vi "Sub Super Duper_8_24_12a_JW.vi"(0 "VISA resource name":refnum<visa-resource-name>="GPIB0::17::INSTR", 1 "Sample Properties:":T6 {"Date Created" format="%<%Y/%m/%d>T"}, 2 "TRF Cluster":T7={"Step 4"=-38.0, "# of Loops"=1.0, "Transfer 2"=FALSE, "Start 4"=-2.0, "Total Points 2"=2, "Start 3"=40.0, "Stop 2"=-40.0, "Step 3"=-1.0, "Loop Step"=0.0, "Integration Time 3"=0, "Loop Wait"=0.0, "First Step"=0.0} {"Loop Wait" format="%<%H:%M:%S>t"; "Integration Time 3" scale=0.0..2.0; "Step 3" format="%.2f"; "Stop 2" format="%.2f"; "Start 3" format="%.2f"; "Start 4" format="%.2f"; "Step 4" format="%.2f"}, 3 "TSP Cluster":T8={"Transport"=FALSE, "Start 2"=0.0, "Stop 3"=-60.0, "Step 2"=-1.0, "Start"=0.0, "Step"=-10.0, "Total Points"=7, "Integration Time"=0} {"Integration Time" scale=0.0..2.0; "Step" format="%.2f"; "Start" format="%.2f"; "Step 2" format="%.2f"; "Stop 3" format="%.2f"; "Start 2" format="%.2f"}, 4 "Compliance Cluster":T3={"Var1 sweep settings"={"sweep spacing (linear: 0)"=0, "sweep mode"=FALSE, "compliance (V)"=100.0, "compliance (A)"=0.001}, "Var1 sweep settings 2"={"sweep spacing (linear: 0)"=0, "sweep mode"=FALSE, "compliance (V)"=100.0, "compliance (A)"=0.001}, "Var2 step settings 2"={"compliance (A)"=0.001, "compliance (V)"=100.0}, "Var2 step settings"={"compliance (A)"=0.001, "compliance (V)"=100.0}} {"Var2 step settings"."compliance (V)" format="%.2f"; "Var2 step settings"."compliance (A)" format="%^.2e"; "Var2 step settings 2"."compliance (V)" format="%.2f"; "Var2 step settings 2"."compliance (A)" format="%^.2e"; "Var1 sweep settings 2"."compliance (A)" format="%^.2e"; "Var1 sweep settings 2"."compliance (V)" format="%.2f"; "Var1 sweep settings 2"."sweep spacing (linear: 0)" items=["linear", "log 10", "log 25", "log 50"]; "Var1 sweep settings"."compliance (A)" format="%^.2e"; "Var1 sweep settings"."compliance (V)" format="%.2f"; "Var1 sweep settings"."sweep spacing (linear: 0)" items=["linear", "log 10", "log 25", "log 50"]}, 5 "error in":errorcluster, 6 "Saved Folder:":path=path "C:/1DATA/2011", 7 "Wait Cluster":T2 {"Wait Time (s)" format="%.1g"; "Wait Countdown" format="%<%H:%M:%S%1u>t"}, 9 "Stop \nCountdown":bool, 11 "Loop Count":dbl) -> (8 "Status Indicator":bool, 10 "Vt Cluster":T1 {"Id Max" format="%.3g"; "Vt Max" format="%.3g"; "Vt Min" format="%.3g"; "Vt Ratio" format="%.3g"}, 14 "VISA resource name out":refnum<visa-resource-name>, 15 "TRF Path":path, 16 "TSP Path":path, 17 "Graph Cluster":T4, 18 "Char Cluster":T5 {"Mobility-Lin" format="%#_4e"; "On/Off" format="%#_4e"; "Mobility-Sat" format="%#_4e"}, 19 "error out":errorcluster)   [LabVIEW 2012]
uses:
  <vilib>/Platform/TimedLoop/XDataNode/wakeup.ctl
  <vilib>/Platform/TimedLoop/XDataNode/XDNodeRunTimeDep.lvlib
  <vilib>/Platform/TimedLoop/XDataNode/nitl_modes.ctl
  <vilib>/Platform/TimedLoop/XDataNode/timing_clust.ctl
  <vilib>/Platform/TimedLoop/XDataNode/XDataNode.xnode
panel:
  # "Vg Sweep"
  # "Vd Step"
  # "Loops and Integration Time"
  # "Device Characteristics"
  # "Sample Properties:"
  # "%"
  # "nm"
  # "Device Properties:"
  # "um"
  # "um"
  # "Vg Step"
  # "Vd Step"
  # "Integration Time"
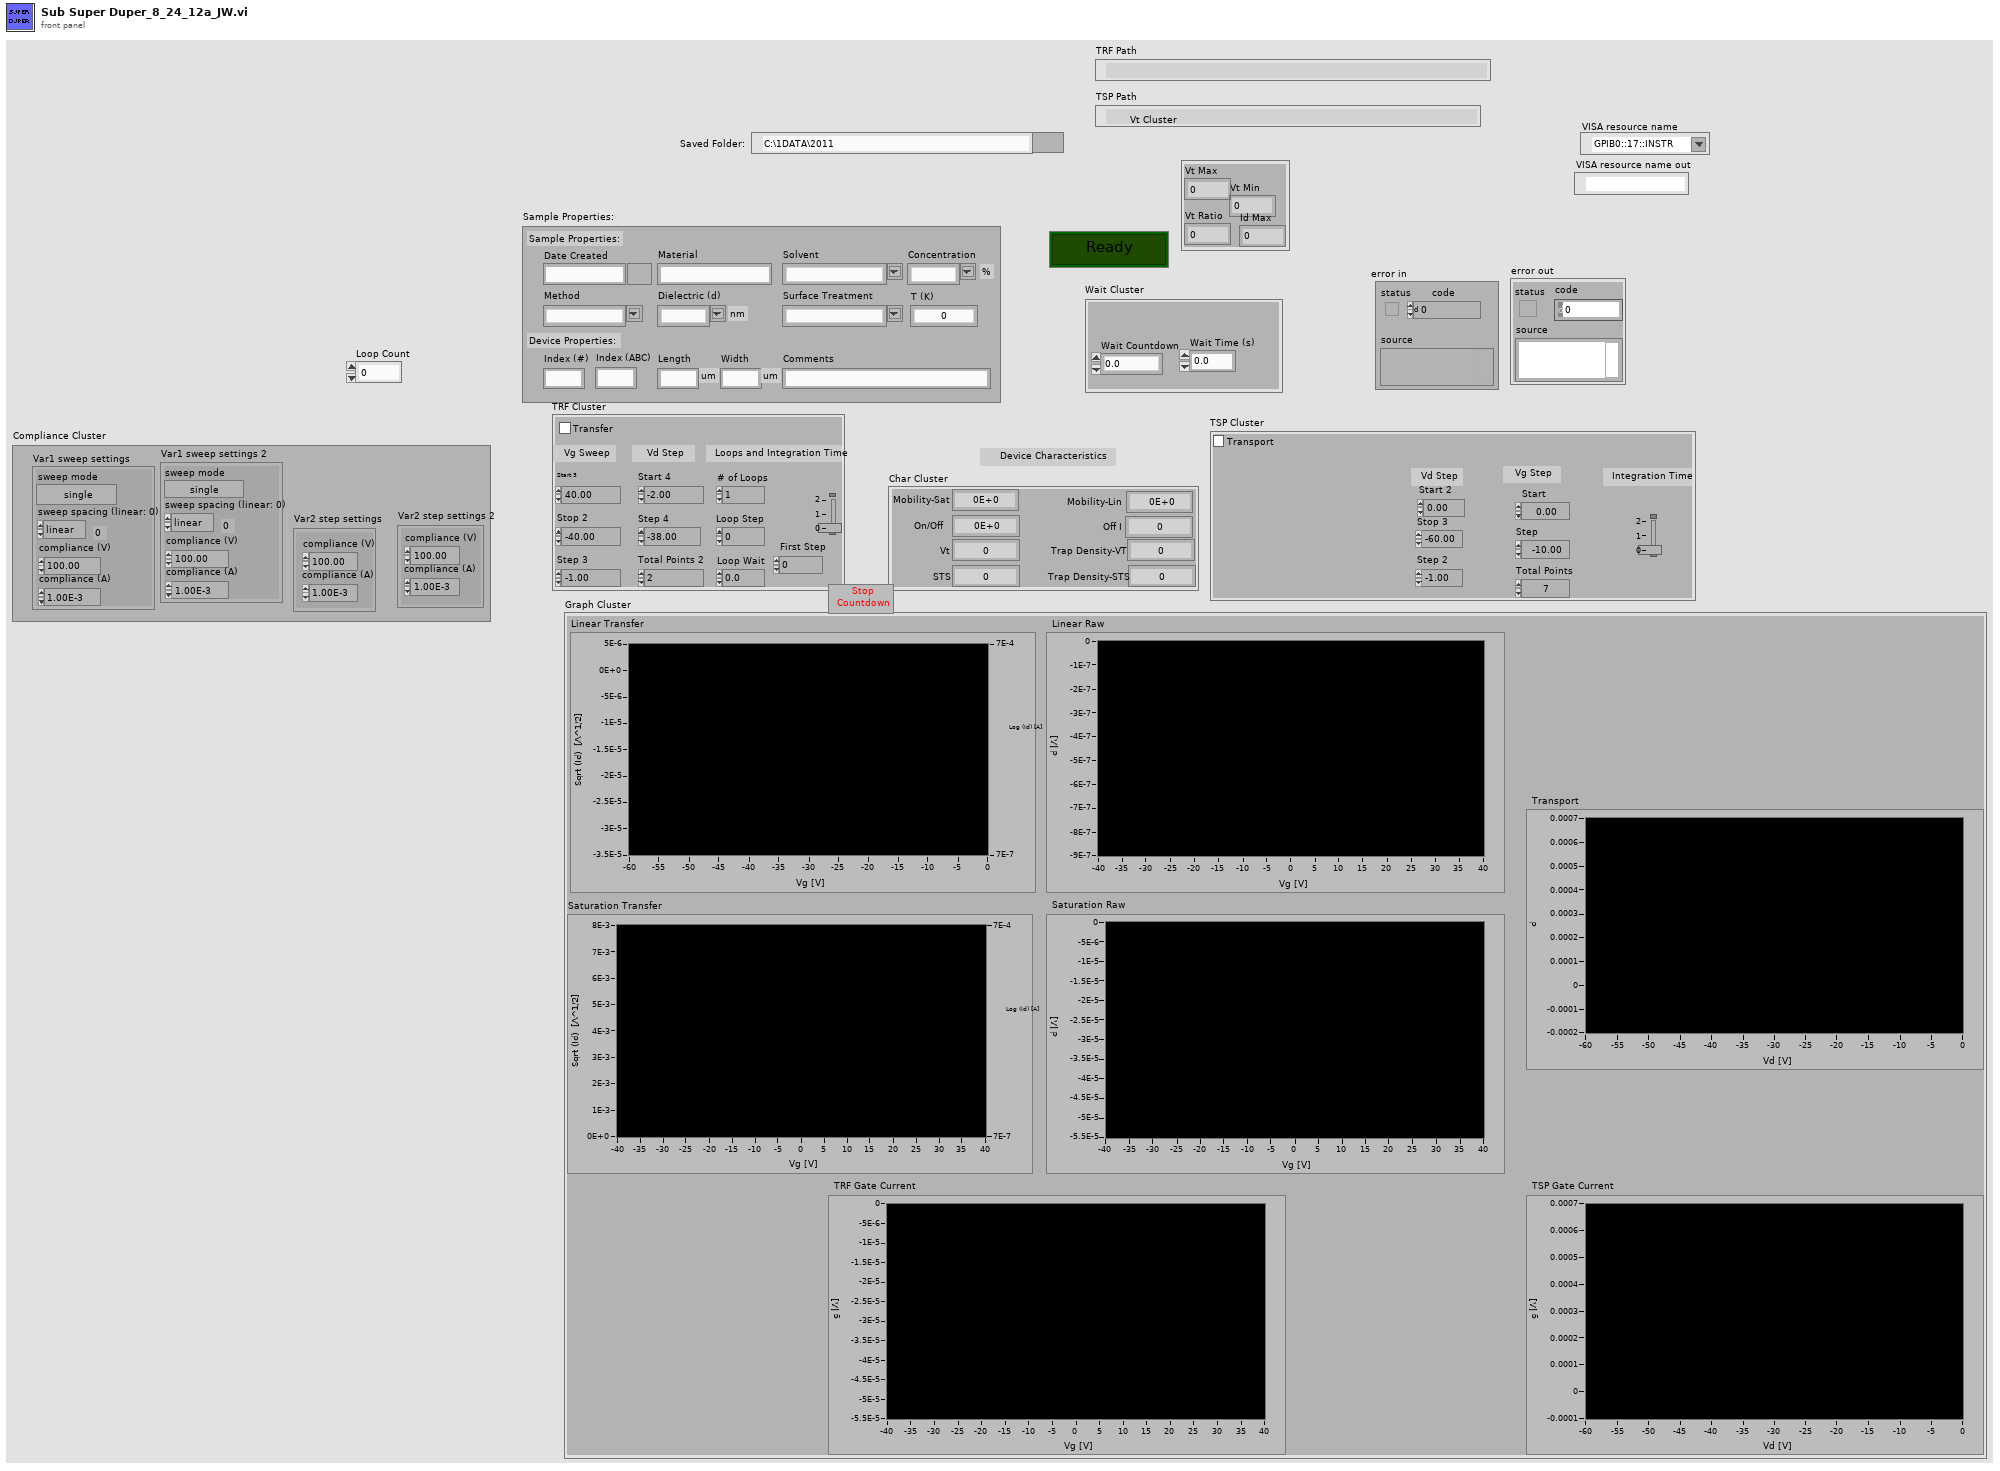
[diagram p1: front panel]
types:
  T1 = cluster{"Vt Max":i32, "Vt Min":i32, "Vt Ratio":i32, "Id Max":i32}
  T2 = cluster{"Wait Countdown":dbl, "Wait Time (s)":dbl}
  T3 = cluster{"Var1 sweep settings":cluster{"sweep spacing (linear: 0)":u16, "sweep mode":bool, "compliance (V)":dbl, "compliance (A)":dbl}, "Var1 sweep settings 2":cluster{"sweep spacing (linear: 0)":u16, "sweep mode":bool, "compliance (V)":dbl, "compliance (A)":dbl}, "Var2 step settings 2":cluster{"compliance (A)":dbl, "compliance (V)":dbl}, "Var2 step settings":cluster{"compliance (A)":dbl, "compliance (V)":dbl}}
  T4 = cluster{"Linear Transfer":cluster{dbl[], "trace":dbl[]}[], "Linear Raw":cluster{dbl[], dbl[]}[], "Saturation Transfer":cluster{dbl[], "trace":dbl[]}[], "Saturation Raw":cluster{dbl[], dbl[]}[], "Transport":cluster{dbl[], dbl[]}[], "TRF Gate Current":cluster{dbl[], dbl[]}[], "TSP Gate Current":cluster{dbl[], dbl[]}[]}
  T5 = cluster{"Mobility-Sat":dbl, "Mobility-Lin":dbl, "On/Off ":dbl, "Off I":dbl, "Vt":dbl, "STS":dbl, "Trap Density-VT":dbl, "Trap Density-STS":dbl}
  T6 = cluster{"Date Created":timestamp, "Material":string, "Solvent":string, "Concentration":string, "Method":string, "Dielectric (d)":string, "Index (#)":string, "Index (ABC)":string, "Length":string, "Width":string, "Surface Treatment":string, "Comments":string, "T (K)":dbl}
  T7 = cluster{"Step 4":dbl, "# of Loops":dbl, "Transfer 2":bool, "Start 4":dbl, "Total Points 2":u16, "Start 3":dbl, "Stop 2":dbl, "Step 3":dbl, "Loop Step":dbl, "Integration Time 3":u32, "Loop Wait":dbl, "First Step":dbl}
  T8 = cluster{"Transport":bool, "Start 2":dbl, "Stop 3":dbl, "Step 2":dbl, "Start":dbl, "Step":dbl, "Total Points":u16, "Integration Time":u32}
  T9 = typedef "XDNodeRunTimeDep.lvlib/timing_clust.ctl" = cluster{"Expected End [f-1]":u64, "Actual End [f-1]":u64, "Finished Late? [f-1]":bool, "Expected End [i-1]":u64, "Actual End [i-1]":u64, "Finished Late? [i-1]":bool, "Expected Start [i]":u64, "Actual Start [i]":u64, "Expected Start [f]":u64, "Actual Start [f]":u64, "Source Name":string, "Structure Name":string, "Period":i64, "Deadline":i64, "Offset":i64, "Start":i64, "Priority":i32, "Timeout":i32, "Mode":T10, "Wakeup Reason":T11, "Error":errorcluster, "Source Type":string, "Secondary Source Type":string, "Global End Time":u64, "Global Start Time":u64, "Frame Duration":u64, "Iteration Duration":u64, "Assigned CPU":i32, "I/O Scan Engine Mode":u32}
  T10 = typedef "XDNodeRunTimeDep.lvlib/nitl_modes.ctl" = enum32{"No Change", "Process missed periods, maintain original phase", "Discard missed periods, maintain original phase", "Process missed periods, ignore original phase", "Discard missed periods, ignore original phase"}
  T11 = typedef "XDNodeRunTimeDep.lvlib/wakeup.ctl" = enum32{"Normal", "Aborted", "Asynchronous wakeup", "Timing source error", "Timed loop error", "Timeout"}
  T12 = cluster{"sweep spacing (linear: 0)":u16, "sweep mode":bool, "compliance (V)":dbl, "compliance (A)":dbl}
  T13 = cluster{"compliance (A)":dbl, "compliance (V)":dbl}
  T14 = cluster{"Start 3":dbl, "Stop 2":dbl, "Step 3":dbl, "sweep spacing (linear: 0)":u16, "sweep mode":bool, "compliance (V)":dbl, "compliance (A)":dbl}
  T15 = cluster{"compliance (A)":dbl, "compliance (V)":dbl, "Start 4":dbl, "Total Points 2":u16, dbl}
  T16 = cluster{"Vt Max":i32, "Vt Min":i32, "Vt Ratio":i32, "Id Max":dbl}
  T17 = cluster{"Mobility-Sat":dbl, "Mobility-Lin":dbl, "On/Off Current":dbl, "Off I":dbl, "Vt":dbl, "STS":dbl, "Trap Density-VT":dbl, "Trap Density-STS":dbl}
  T18 = cluster{"Linear Sqrt":cluster{dbl[], "trace":dbl[]}[], "Linear Log":cluster{dbl[], "trace":dbl[]}[], "Linear Raw":cluster{dbl[], dbl[]}[], "Saturation Sqrt":cluster{dbl[], "trace":dbl[]}[], "Saturation Log":cluster{dbl[], "trace":dbl[]}[], "Saturation Raw":cluster{dbl[], "trace":dbl[]}[], "Gate Current":cluster{dbl[], "trace":dbl[]}[]}
  T19 = cluster{"Start 2":dbl, "Stop 3":dbl, "Step 2":dbl, "sweep spacing (linear: 0)":u16, "sweep mode":bool, "compliance (V)":dbl, "compliance (A)":dbl}
  T20 = cluster{"compliance (A)":dbl, "compliance (V)":dbl, "Start":dbl, "Total Points":u16, "Step":dbl}
  T21 = cluster{"Transport":cluster{dbl[], dbl[]}[], "Gate Current":cluster{dbl[], dbl[]}[]}
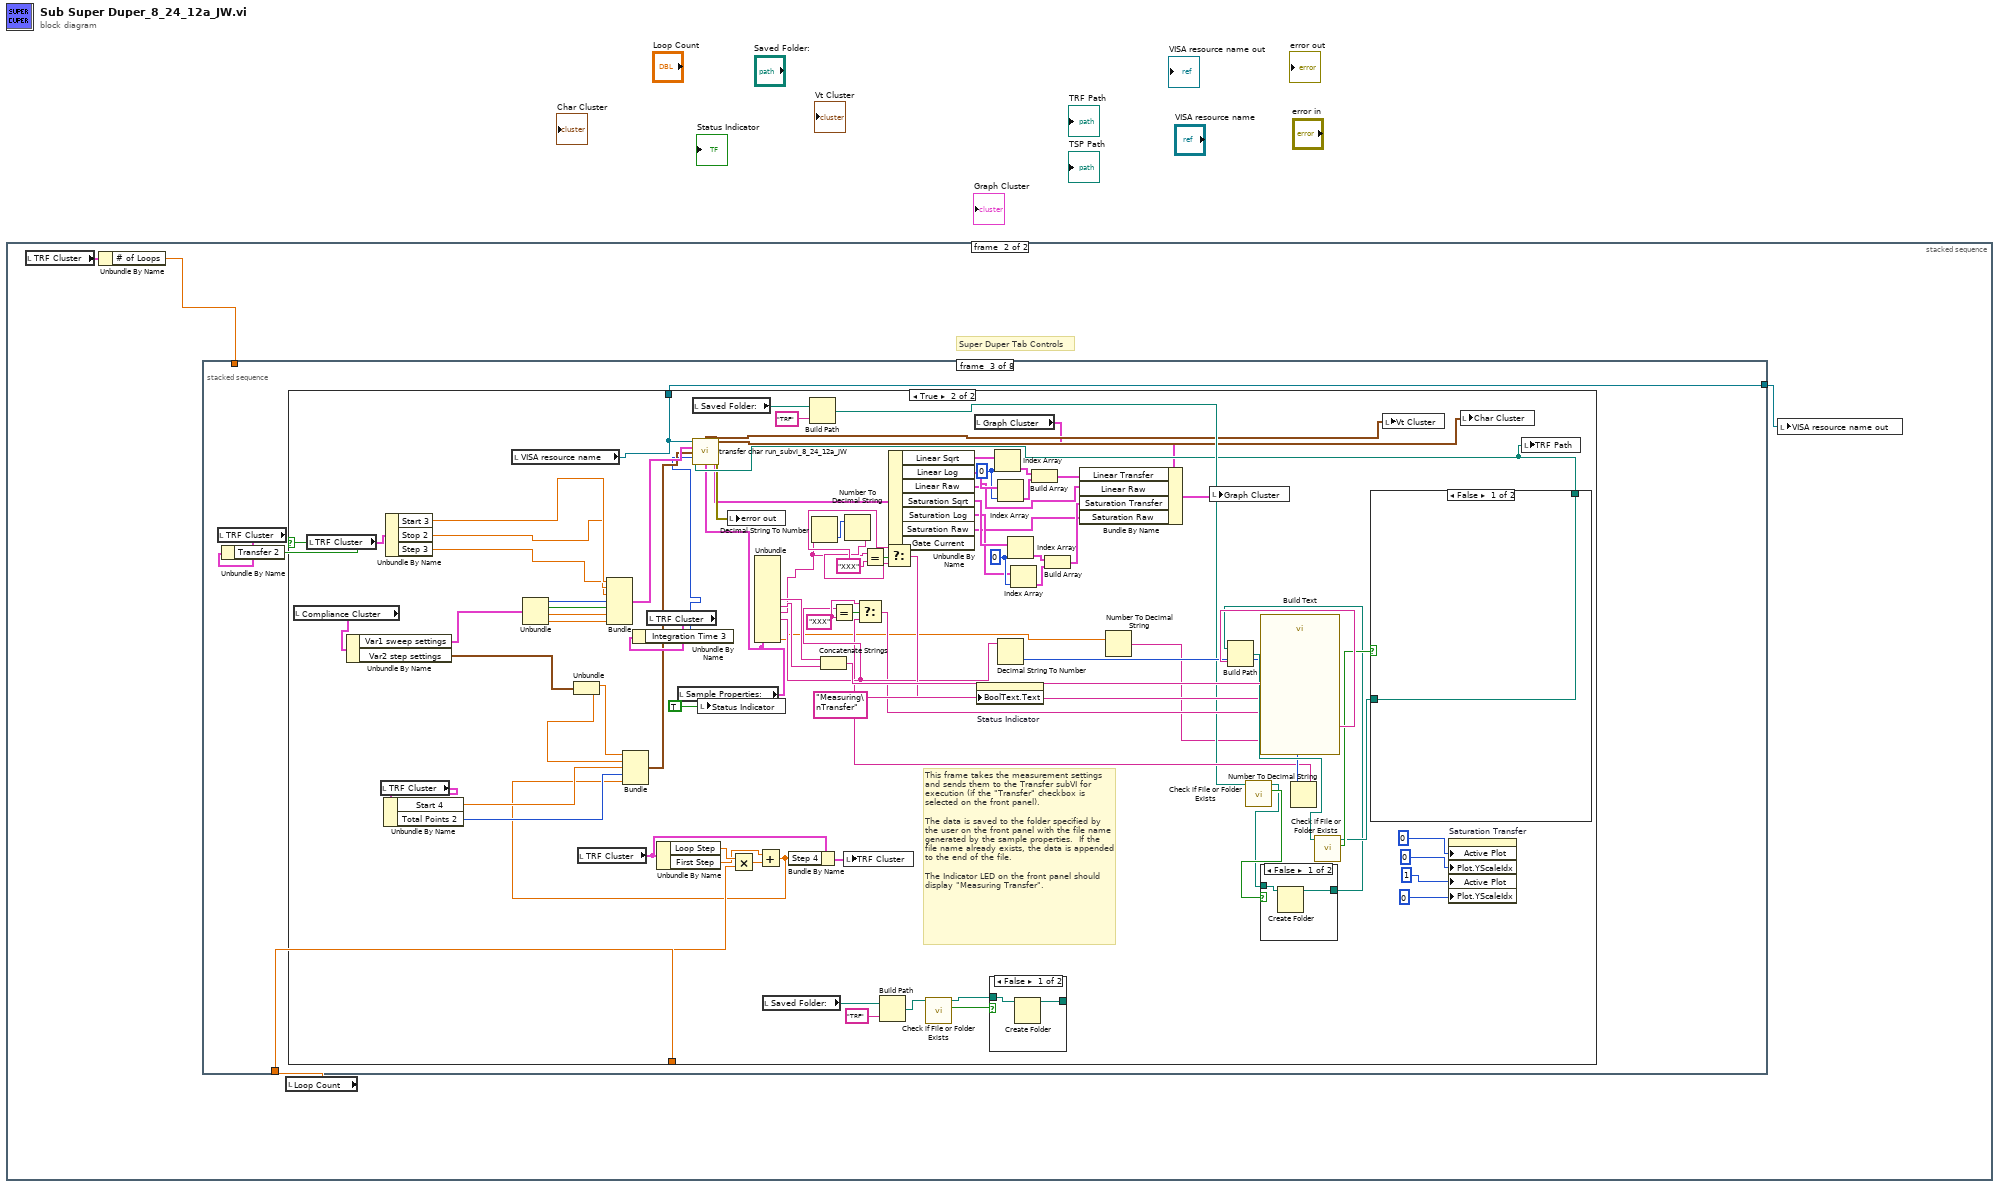
[diagram p0: block diagram]
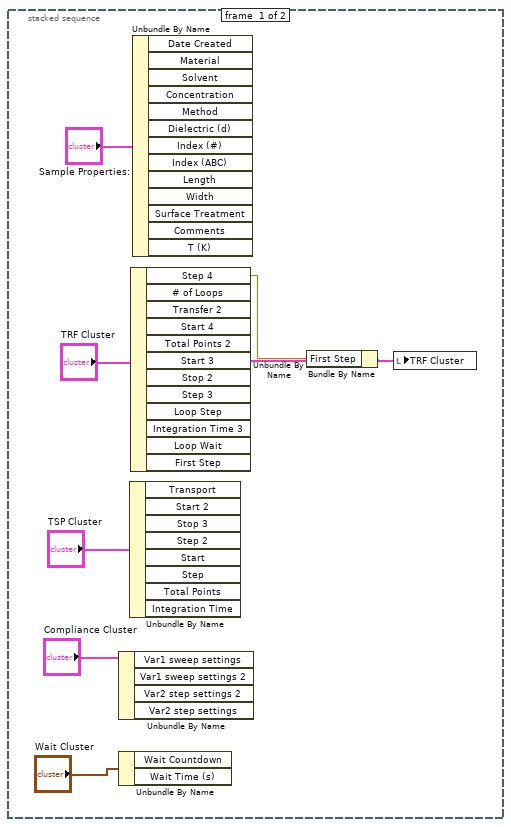
[diagram p2: hidden frame]
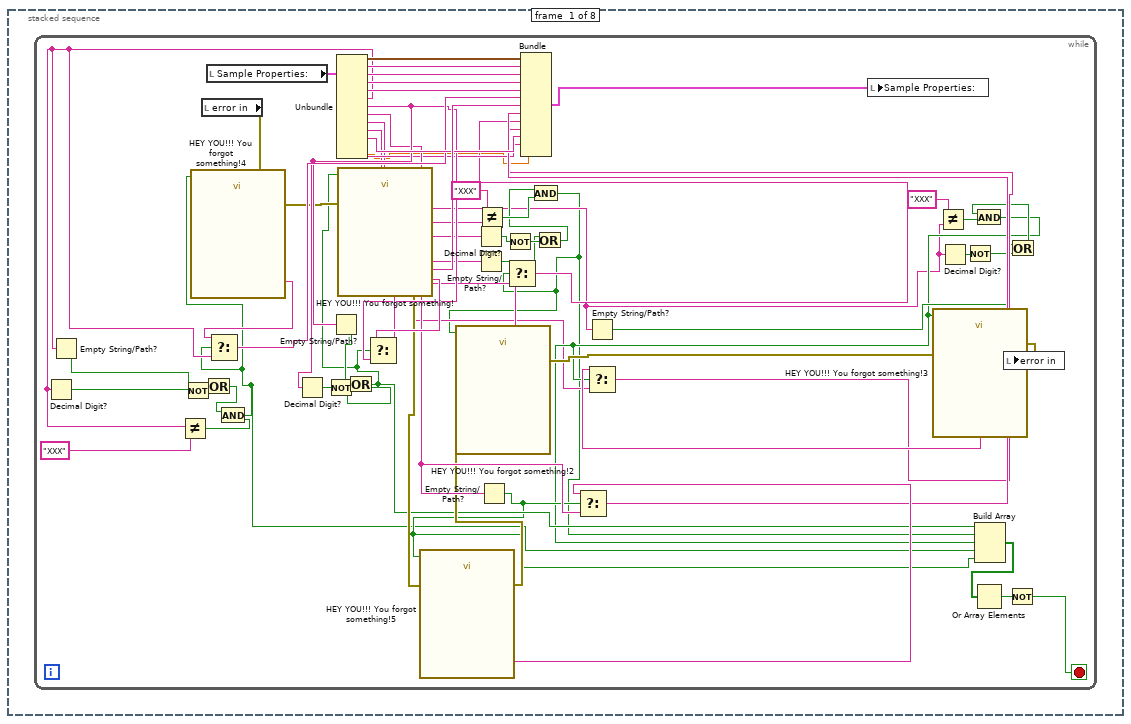
[diagram p3: hidden frame]
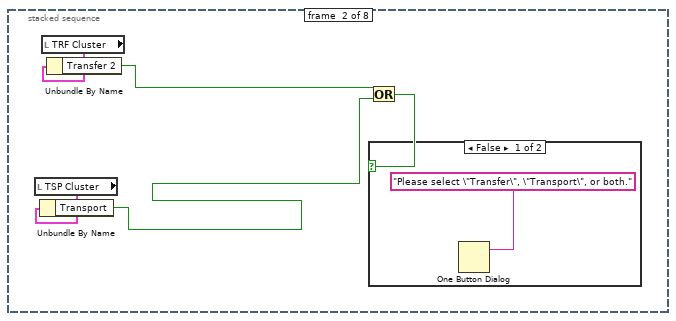
[diagram p4: hidden frame]
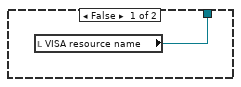
[diagram p6: hidden frame]
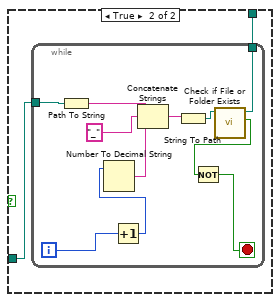
[diagram p9: hidden frame]
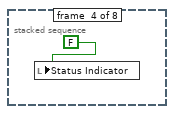
[diagram p10: hidden frame]
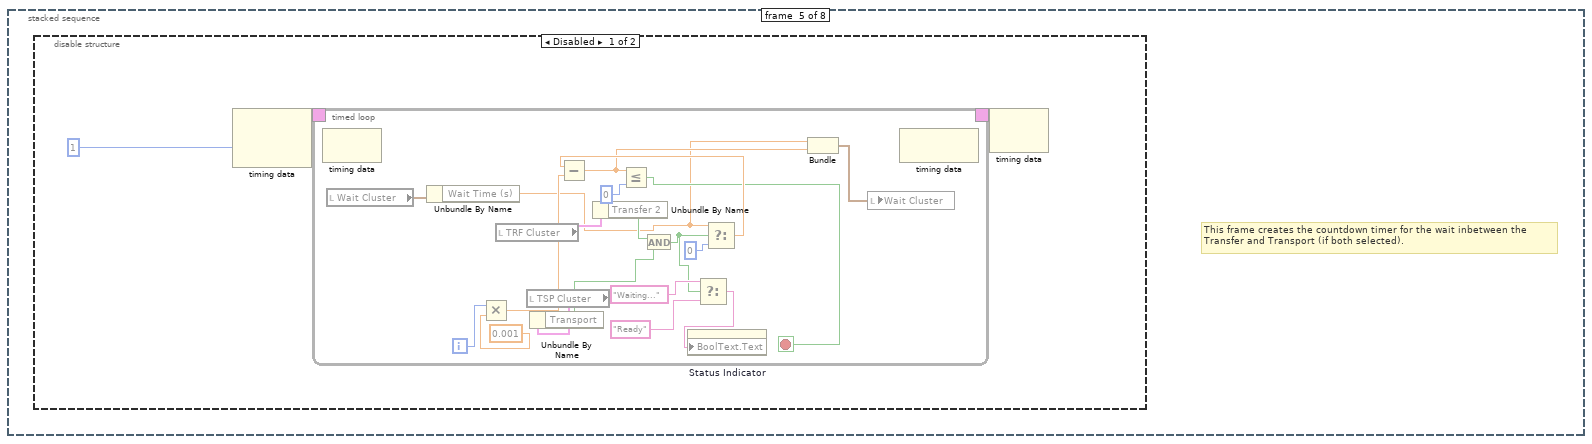
[diagram p11: hidden frame]
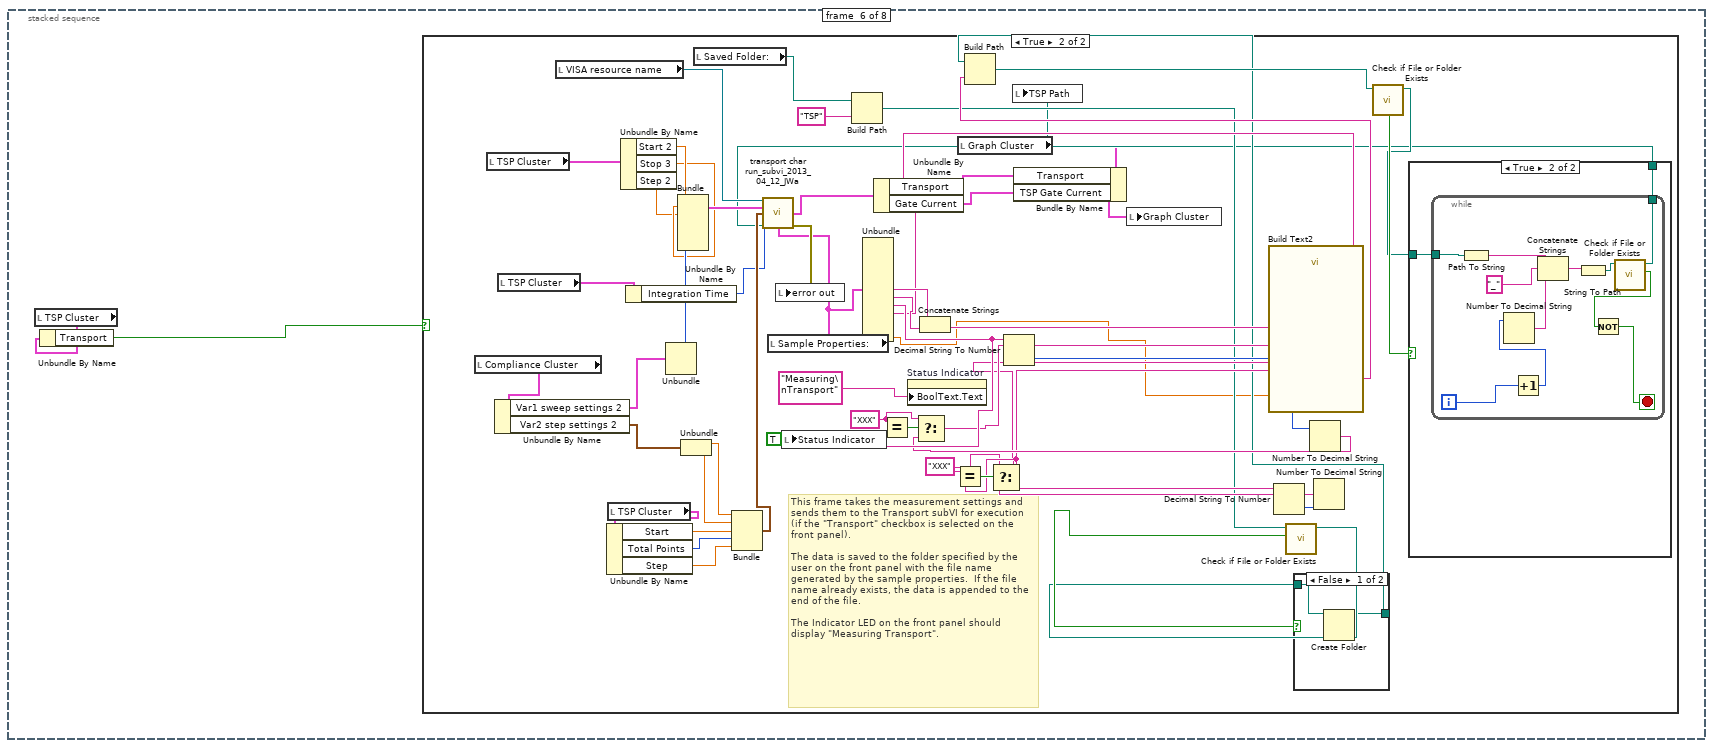
[diagram p13: hidden frame]
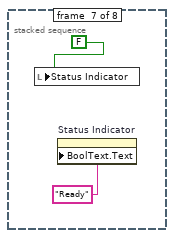
[diagram p17: hidden frame]
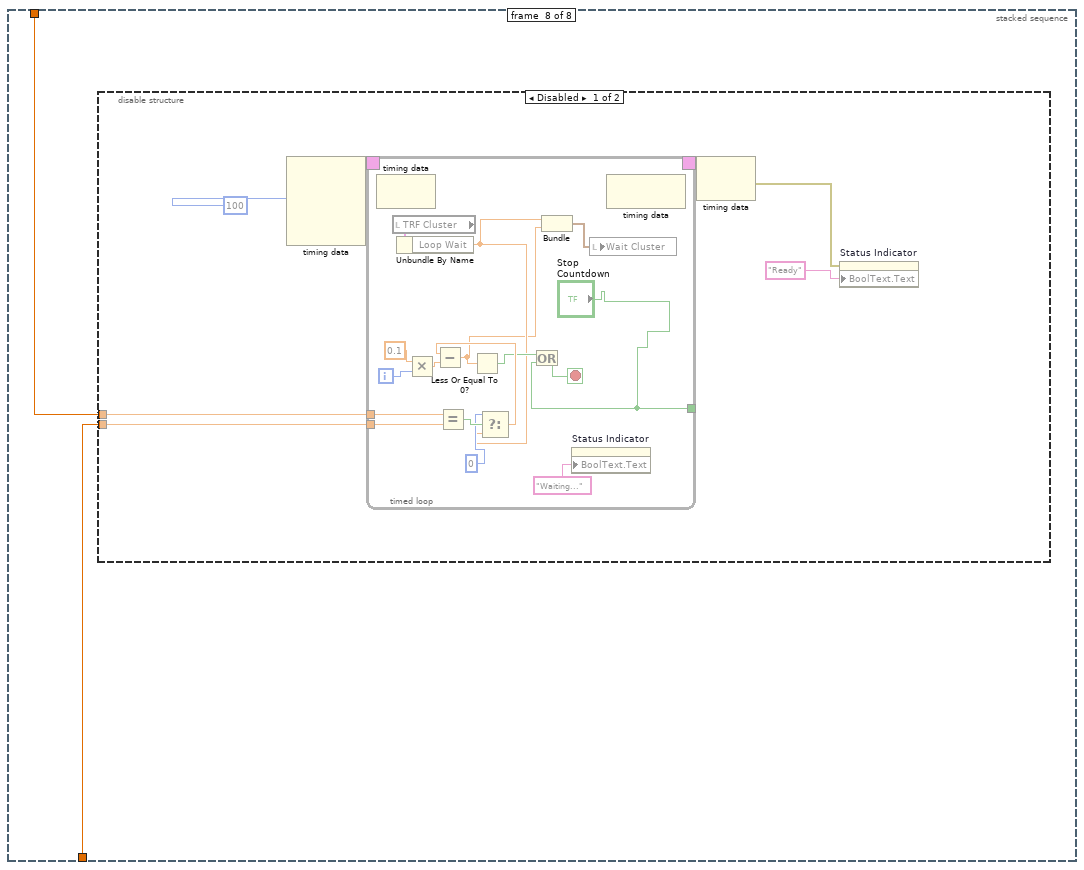
[diagram p18: hidden frame]
diagram:
  n1 = stacked-sequence {
    frame #0 {
      n2 = Unbundle By Name("Compliance Cluster") -> ()  [unwired: 4 out]
      n3 = Unbundle By Name("Wait Cluster") -> ()  [unwired: 2 out]
      n4 = Unbundle By Name("TSP Cluster") -> ()  [unwired: 8 out]
      n5 = Unbundle By Name("TRF Cluster") -> ("Step 4"=w7:dbl)  [unwired: 11 out]
      n6 = Unbundle By Name("Sample Properties:") -> ()  [unwired: 13 out]
      n7 = Bundle By Name(cluster="TRF Cluster", "First Step"=w7) -> (w5:T7)
      n8 = local write "TRF Cluster"(w5) -> ()
    }
    frame #1 {
      # "Super Duper Tab Controls"
      n9 = local read "TRF Cluster"() -> (w11:T7)
      n10 = Unbundle By Name(w11) -> ("# of Loops"=w10:dbl)
      n11 = local read "Loop Count"() -> (w8:dbl)
      n12 = stacked-sequence {
        tunnel: w8 -> [_ _ w81 _ _ _ _ w300]
        tunnel: w10 -> [_ _ _ _ _ _ _ w299]
        tunnel: [_ _ w78 _ _ _ _ _] -> w9
        frame #0 {
          n13 = while {
            stop <- w37 stop-if-true
            n14 = local read "error in"() -> (w43:errorcluster)
            n15 = local read "Sample Properties:"() -> (w66:T6)
            n16 = Unbundle(w66) -> ("Date Created"=w67:timestamp, "Material"=w68:string, "Solvent"=w69:string, "Concentration"=w70:string, "Method"=w71:string, "Dielectric (d)"=w26:string, "Index (#)"=w56:string, "Index (ABC)"=w53:string, "Length"=w21:string, "Width"=w14:string, "Surface Treatment"=w59:string, "Comments"=w51:string, "T (K)"=w12:dbl)
            n17 = Decimal Digit?(1:w26) -> (0:w34:bool)
            n18 = Empty String/Path?(string/path=w26) -> (empty?=w28:bool)
            n19 = Not Equal?(x=w26, y="XXX") -> (x != y?=w25:bool)
            n20 = Not(x=w34) -> (.not. x?=w31:bool)
            n21 = Or(x=w28, y=w31) -> (x .or. y?=w24:bool)
            n22 = And(x=w24, y=w25) -> (x .and. y?=w23:bool)
            n23 = call "HEY YOU!!! You forgot something!4"("Enable"=w23, "error in (no error)"=w43) -> ("Dielectric (d)"=w58:string, "error out"=w42:errorcluster)  [unwired: 15 in, 1 out]
            n24 = Select(t=w58, s=w23, f=w26) -> (s? t:f=w57:string)
            n25 = Decimal Digit?(1:w56) -> (0:w47:bool)
            n26 = Not(x=w47) -> (.not. x?=w46:bool)
            n27 = Empty String/Path?(string/path=w56) -> (empty?=w55:bool)
            n28 = Or(x=w55, y=w46) -> (x .or. y?=w41:bool)
            n29 = call "HEY YOU!!! You forgot something!"("Enable"=w41, "error in (no error)"=w42) -> ("Index (#)"=w65:string, "error out"=w45:errorcluster)  [unwired: 15 in, 1 out]
            n30 = Select(t=w65, s=w41, f=w56) -> (s? t:f=w62:string)
            n31 = Decimal Digit?(1:w21) -> (0:w36:bool)
            n32 = Empty String/Path?(string/path=w21) -> (empty?=w30:bool)
            n33 = Not Equal?(x="XXX", y=w21) -> (x != y?=w20:bool)
            n34 = Empty String/Path?(string/path=w53) -> (empty?=w40:bool)
            n35 = call "HEY YOU!!! You forgot something!5"("Enable"=w40, "error in (no error)"=w45) -> ("Index (ABC)"=w54:string, "error out"=w44:errorcluster)  [unwired: 15 in, 1 out]
            n36 = Not(x=w36) -> (.not. x?=w33:bool)
            n37 = Or(x=w30, y=w33) -> (x .or. y?=w19:bool)
            n38 = And(x=w19, y=w20) -> (x .and. y?=w13:bool)
            n39 = call "HEY YOU!!! You forgot something!2"("Enable"=w13, "error in (no error)"=w44) -> ("Length"=w64:string, "error out"=w61:errorcluster)  [unwired: 15 in, 1 out]
            n40 = Select(t=w64, s=w13, f=w21) -> (s? t:f=w50:string)
            n41 = Select(t=w54, s=w40, f=w53) -> (s? t:f=w52:string)
            n42 = Empty String/Path?(string/path=w14) -> (empty?=w29:bool)
            n43 = Not Equal?(x="XXX", y=w14) -> (x != y?=w18:bool)
            n44 = Decimal Digit?(1:w14) -> (0:w35:bool)
            n45 = Not(x=w35) -> (.not. x?=w32:bool)
            n46 = Or(x=w29, y=w32) -> (x .or. y?=w17:bool)
            n47 = And(x=w17, y=w18) -> (x .and. y?=w16:bool)
            n48 = call "HEY YOU!!! You forgot something!3"("Enable"=w16, "error in (no error)"=w61) -> ("Width"=w63:string, "error out"=w60:errorcluster)  [unwired: 15 in, 1 out]
            n49 = Select(t=w63, s=w16, f=w14) -> (s? t:f=w49:string)
            n50 = Bundle("Date Created"=w67, "Material"=w68, "Solvent"=w69, "Concentration"=w70, "Method"=w71, "Dielectric (d)"=w57, "Index (#)"=w62, "Index (ABC)"=w52, "Length"=w50, "Width"=w49, "Surface Treatment"=w59, "Comments"=w51, "T (K)"=w12) -> (w48:T6)  [unwired: 1 in]
            n51 = local write "Sample Properties:"(w48) -> ()
            n52 = Build Array(w41, w13, w16, w23, w40) -> (w39:bool[])
            n53 = Or Array Elements(Boolean array=w39) -> (logical OR=w38:bool)
            n54 = local write "error in"(w60) -> ()
            n55 = Not(x=w38) -> (.not. x?=w37:bool)
          }
        }
        frame #1 {
          n56 = local read "TSP Cluster"() -> (w73:T8)
          n57 = Unbundle By Name(w73) -> ("Transport"=w72:bool)
          n58 = local read "TRF Cluster"() -> (w75:T7)
          n59 = Unbundle By Name(w75) -> ("Transfer 2"=w74:bool)
          n60 = Or(x=w74, y=w72) -> (x .or. y?=w76:bool)
          n61 = case shown="False" w76 {
            frame False {
              n62 = One Button Dialog(message="Please select \"Transfer\", \"Transport\", or both.") -> ()  [unwired: 1 in, 1 out]
            }
            frame True {
            }
          }
        }
        frame #2 {
          n63 = local read "TRF Cluster"() -> (w79:T7)
          n64 = Unbundle By Name(w79) -> ("Transfer 2"=w80:bool)
          n65 = case shown="True" w80 {
            tunnel: w81 -> [_ w119]
            tunnel: [w82 w113] -> w78
            frame False {
              n66 = local read "VISA resource name"() -> (w82:refnum<visa-resource-name>)
            }
            frame True {
              w94 = 0
              w100 = 0
              w148 = "XXX"
              w152 = "XXX"
              # "This frame takes the measurement settings and sends them to the Transfer subVI for execution (if the \"Transfer\" checkbox is selected on the front panel).\n\nThe data is saved to the folder specified by the user on the front panel with the file name generated by the sample properties.  If the file name already exists, the data is appended to the end of the file.\n\nThe Indicator LED on the front panel should display \"Measuring Transfer\"."
              n67 = local read "Compliance Cluster"() -> (w125:T3)
              n68 = local read "TRF Cluster"() -> (w131:T7)
              n69 = Unbundle By Name(w125) -> ("Var1 sweep settings"=w123:T12, "Var2 step settings"=w124:T13)
              n70 = local read "TRF Cluster"() -> (w134:T7)
              n71 = Unbundle By Name(w134) -> ("Start 4"=w133:dbl, "Total Points 2"=w132:u16)
              n72 = Unbundle By Name(w131) -> ("Start 3"=w130:dbl, "Stop 2"=w129:dbl, "Step 3"=w128:dbl)
              n73 = local read "VISA resource name"() -> (w113:refnum<visa-resource-name>)
              n74 = Unbundle(w123) -> ("sweep spacing (linear: 0)"=w170:u16, "sweep mode"=w169:bool, "compliance (V)"=w168:dbl, "compliance (A)"=w167:dbl)
              n75 = Unbundle(w124) -> ("compliance (A)"=w166:dbl, "compliance (V)"=w165:dbl)
              n76 = local read "TRF Cluster"() -> (w114:T7)
              n77 = Bundle("Start 3"=w130, "Stop 2"=w129, "Step 3"=w128, "sweep spacing (linear: 0)"=w170, "sweep mode"=w169, "compliance (V)"=w168, "compliance (A)"=w167) -> (w112:T14)  [unwired: 1 in]
              n78 = local read "TRF Cluster"() -> (w127:T7)
              n79 = Unbundle By Name(w127) -> ("Integration Time 3"=w110:u32)
              n80 = Unbundle By Name(w114) -> ("Loop Step"=w117:dbl, "First Step"=w116:dbl)
              n81 = local read "Sample Properties:"() -> (w108:T6)
              n82 = local read "Saved Folder:"() -> (w126:path)
              n83 = local write "Status Indicator"(TRUE) -> ()
              n84 = Multiply(x=w117, y=w119) -> (x*y=w120:dbl)
              n85 = Unbundle(w108) -> ("Index (#)"=w161:string, "Index (ABC)"=w160:string, "Length"=w144:string, "Width"=w147:string, "T (K)"=w122:dbl)  [unwired: 8 out]
              n86 = Add(x=w116, y=w120) -> (x+y=w115:dbl)
              n87 = Bundle("compliance (A)"=w166, "compliance (V)"=w165, "Start 4"=w133, "Total Points 2"=w132, w115) -> (w111:T15)  [unwired: 1 in]
              n88 = local read "Saved Folder:"() -> (w87:path)
              n89 = Bundle By Name(cluster=w114, "Step 4"=w115) -> (w118:T7)
              n90 = Build Path(base path=w126, name or relative path="TRF") -> (appended path=w140:path)
              n91 = Decimal String To Number(string=w144) -> (number=w155:i32)  [unwired: 2 in, 1 out]
              n92 = Concatenate Strings(w161, w160) -> (w159:string)
              n93 = Equal?(x=w147, y=w148) -> (x = y?=w149:bool)
              n94 = local write "TRF Cluster"(w118) -> ()
              n95 = Number To Decimal String(number=w155) -> (decimal integer string=w151:string)  [unwired: 1 in]
              n96 = Equal?(x=w144, y=w152) -> (x = y?=w153:bool)
              n97 = Build Path(base path=w87, name or relative path="TRF") -> (appended path=w85:path)
              n98 = Select(t=w152, s=w153, f=w151) -> (s? t:f=w150:string)
              n99 = call <vilib>:"Check if File or Folder Exists.vi"("path"=w85) -> ("file or folder exists?"=w83:bool, "dup path"=w84:path)  [unwired: 8 in, 1 out]
              n100 = local read "Graph Cluster"() -> (w103:T4)
              n101 = property on="Status Indicator" class="Bool (strict)"("BoolText.Text"="Measuring\nTransfer") -> ()  [unwired: 2 in, 2 out]
              n102 = case shown="False" w83 {
                tunnel: w84 -> [w172 w173]
                tunnel: [w171 w173] -> _
                frame False {
                  n103 = Create Folder(path (use dialog)=w172) -> (created path=w171:path)  [unwired: 2 in, 2 out]
                }
                frame True {
                }
              }
              n104 = Decimal String To Number(string=w147) -> (number=w154:i32)  [unwired: 2 in, 1 out]
              n105 = Number To Decimal String(number=w122) -> (decimal integer string=w121:string)  [unwired: 1 in]
              n106 = call <vilib>:"Check if File or Folder Exists.vi"("path"=w140) -> ("file or folder exists?"=w142:bool, "dup path"=w141:path)  [unwired: 8 in, 1 out]
              n107 = case shown="False" w142 {
                tunnel: w141 -> [w175 w176]
                tunnel: [w174 w176] -> w139
                frame False {
                  n108 = Create Folder(path (use dialog)=w175) -> (created path=w174:path)  [unwired: 2 in, 2 out]
                }
                frame True {
                }
              }
              n109 = Number To Decimal String(number=w154) -> (decimal integer string=w146:string)  [unwired: 1 in]
              n110 = Select(t=w148, s=w149, f=w146) -> (s? t:f=w145:string)
              n111 = call "Build Text"("T"=w121, "Index"=w159, "Length"=w150, "Width"=w145) -> ("Result"=w164:string)  [unwired: 10 in, 1 out]
              n112 = Build Path(base path=w139, name or relative path=w164) -> (appended path=w157:path)
              n113 = call <vilib>:"Check if File or Folder Exists.vi"("path"=w157) -> ("file or folder exists?"=w158:bool, "dup path"=w156:path)  [unwired: 8 in, 1 out]
              n114 = case shown="False" w158 {
                tunnel: w156 -> [w177 w179]
                tunnel: [w177 w178] -> w109
                frame False {
                }
                frame True {
                  n115 = while {
                    tunnel: w179 -> [w181]
                    tunnel: [w180] -> w178
                    i -> [w183]
                    stop <- w184 stop-if-true
                    n116 = Path To String(path=w181) -> (string=w190:string)
                    n117 = Increment(x=w183) -> (x+1=w182:i32)
                    n118 = Number To Decimal String(number=w182) -> (decimal integer string=w188:string)  [unwired: 1 in]
                    n119 = Concatenate Strings(w190, "_", w188) -> (w187:string)
                    n120 = String To Path(string=w187) -> (path=w186:path)
                    n121 = call <vilib>:"Check if File or Folder Exists.vi"("path"=w186) -> ("file or folder exists?"=w185:bool, "dup path"=w180:path)  [unwired: 8 in, 1 out]
                    n122 = Not(x=w185) -> (.not. x?=w184:bool)
                  }
                }
              }
              n123 = call "transfer char run_subvi_8_24_12a_JW.vi"("VISA session"=w113, "Var1 sweep settings"=w112, "Var2 step settings"=w111, "integration time"=w110, "Input Path"=w109, "Sample Properties:"=w108) -> ("Check Cluster"=w105:T16, "Output"=w106:T17, "Graph Cluster"=w104:T18, "error?"=w107:errorcluster)  [unwired: 6 in]
              n124 = local write "error out"(w107) -> ()
              n125 = Unbundle By Name(w104) -> ("Linear Sqrt"=w102:cluster{dbl[], "trace":dbl[]}[], "Linear Log"=w101:cluster{dbl[], "trace":dbl[]}[], "Linear Raw"=w90:cluster{dbl[], dbl[]}[], "Saturation Sqrt"=w93:cluster{dbl[], "trace":dbl[]}[], "Saturation Log"=w92:cluster{dbl[], "trace":dbl[]}[], "Saturation Raw"=w89:cluster{dbl[], "trace":dbl[]}[])  [unwired: 1 out]
              n126 = Index Array(array=w102, index=w100) -> (element=w99:cluster{dbl[], "trace":dbl[]})
              n127 = Index Array(array=w101, index=w100) -> (element=w98:cluster{dbl[], "trace":dbl[]})
              n128 = Index Array(array=w93, index=w94) -> (element=w95:cluster{dbl[], "trace":dbl[]})
              n129 = Index Array(array=w92, index=w94) -> (element=w96:cluster{dbl[], "trace":dbl[]})
              n130 = Build Array(w99, w98) -> (w97:cluster{dbl[], "trace":dbl[]}[])
              n131 = Build Array(w95, w96) -> (w91:cluster{dbl[], "trace":dbl[]}[])
              n132 = Bundle By Name(cluster=w103, "Linear Transfer"=w97, "Linear Raw"=w90, "Saturation Transfer"=w91, "Saturation Raw"=w89) -> (w88:T4)
              n133 = local write "Graph Cluster"(w88) -> ()
              n134 = local write "Vt Cluster"(w105) -> ()
              n135 = property on="Saturation Transfer" class="XYGraph (strict)"("Active Plot"=0, "Plot.YScaleIdx"=0, "Active Plot"=1, "Plot.YScaleIdx"=0) -> ()  [unwired: 2 in, 2 out]
              n136 = local write "Char Cluster"(w106) -> ()
              n137 = local write "TRF Path"(w109) -> ()
            }
          }
        }
        frame #3 {
          n138 = local write "Status Indicator"(FALSE) -> ()
        }
        frame #4 {
          # "This frame creates the countdown timer for the wait inbetween the\nTransfer and Transport (if both selected)."
          n139 = disable-structure shown="Disabled" {
            frame Disabled {
              n140 = node-c288(1) -> (w194:T9)  [unwired: 1 in]
              n141 = timed-loop {
                timing: w194 -> [_]
                timing-out: [_] -> w193
                i -> [w205]
                stop <- w206 stop-if-true
                n142 = node-c288() -> ()  [unwired: 1 in, 1 out]
                n143 = local read "Wait Cluster"() -> (w198:T2)
                n144 = Unbundle By Name(w198) -> ("Wait Time (s)"=w196:dbl)
                n145 = Multiply(x=w205, y=0.001) -> (x*y=w203:dbl)
                n146 = local read "TRF Cluster"() -> (w199:T7)
                n147 = local read "TSP Cluster"() -> (w200:T8)
                n148 = Unbundle By Name(w200) -> ("Transport"=w201:bool)
                n149 = Unbundle By Name(w199) -> ("Transfer 2"=w202:bool)
                n150 = And(x=w202, y=w201) -> (x .and. y?=w210:bool)
                n151 = Select(t="Waiting...", s=w210, f="Ready") -> (s? t:f=w212:string)
                n152 = property on="Status Indicator" class="Bool (strict)"("BoolText.Text"=w212) -> ()  [unwired: 2 in, 2 out]
                n153 = Select(t=w196, s=w210, f=0) -> (s? t:f=w208:dbl)
                n154 = Subtract(x=w208, y=w203) -> (x-y=w197:dbl)
                n155 = Less Or Equal?(x=w197, y=0) -> (x <= y?=w206:bool)
                n156 = Bundle("Wait Time (s)"=w196, w197) -> (w195:cluster{"Wait Time (s)":dbl, dbl})  [unwired: 1 in]
                n157 = local write "Wait Cluster"(w195) -> ()
                n158 = node-c288() -> ()  [unwired: 1 in, 1 out]
              }
              n159 = node-c288(w193) -> ()  [unwired: 1 out]
            }
            frame Enabled {
            }
          }
        }
        frame #5 {
          n160 = local read "TSP Cluster"() -> (w221:T8)
          n161 = Unbundle By Name(w221) -> ("Transport"=w220:bool)
          n162 = case shown="True" w220 {
            frame False {
            }
            frame True {
              w252 = "XXX"
              w256 = "XXX"
              # "This frame takes the measurement settings and sends them to the Transport subVI for execution (if the \"Transport\" checkbox is selected on the front panel).\n\nThe data is saved to the folder specified by the user on the front panel with the file name generated by the sample properties.  If the file name already exists, the data is appended to the end of the file.\n\nThe Indicator LED on the front panel should display \"Measuring Transport\"."
              n163 = local read "Compliance Cluster"() -> (w231:T3)
              n164 = local read "TSP Cluster"() -> (w243:T8)
              n165 = Unbundle By Name(w231) -> ("Var1 sweep settings 2"=w230:T12, "Var2 step settings 2"=w229:T13)
              n166 = local read "TSP Cluster"() -> (w236:T8)
              n167 = local read "VISA resource name"() -> (w233:refnum<visa-resource-name>)
              n168 = local read "TSP Cluster"() -> (w234:T8)
              n169 = Unbundle By Name(w234) -> ("Start"=w239:dbl, "Total Points"=w238:u16, "Step"=w237:dbl)
              n170 = Unbundle By Name(w243) -> ("Start 2"=w242:dbl, "Stop 3"=w241:dbl, "Step 2"=w240:dbl)
              n171 = Unbundle By Name(w236) -> ("Integration Time"=w235:u32)
              n172 = Unbundle(w230) -> ("sweep spacing (linear: 0)"=w279:u16, "sweep mode"=w278:bool, "compliance (V)"=w277:dbl, "compliance (A)"=w276:dbl)
              n173 = Bundle("Start 2"=w242, "Stop 3"=w241, "Step 2"=w240, "sweep spacing (linear: 0)"=w279, "sweep mode"=w278, "compliance (V)"=w277, "compliance (A)"=w276) -> (w275:T19)  [unwired: 1 in]
              n174 = Unbundle(w229) -> ("compliance (A)"=w274:dbl, "compliance (V)"=w273:dbl)
              n175 = local read "Saved Folder:"() -> (w232:path)
              n176 = Bundle("compliance (A)"=w274, "compliance (V)"=w273, "Start"=w239, "Total Points"=w238, "Step"=w237) -> (w272:T20)  [unwired: 1 in]
              n177 = local read "Sample Properties:"() -> (w268:T6)
              n178 = local write "Status Indicator"(TRUE) -> ()
              n179 = Build Path(base path=w232, name or relative path="TSP") -> (appended path=w245:path)
              n180 = Unbundle(w268) -> ("Index (#)"=w267:string, "Index (ABC)"=w266:string, "Length"=w257:string, "Width"=w253:string, "T (K)"=w227:dbl)  [unwired: 8 out]
              n181 = Equal?(x=w256, y=w257) -> (x = y?=w258:bool)
              n182 = property on="Status Indicator" class="Bool (strict)"("BoolText.Text"="Measuring\nTransport") -> ()  [unwired: 2 in, 2 out]
              n183 = Concatenate Strings(w267, w266) -> (w265:string)
              n184 = Equal?(x=w252, y=w253) -> (x = y?=w261:bool)
              n185 = local read "Graph Cluster"() -> (w225:T4)
              n186 = Decimal String To Number(string=w257) -> (number=w260:i32)  [unwired: 2 in, 1 out]
              n187 = Decimal String To Number(string=w253) -> (number=w259:i32)  [unwired: 2 in, 1 out]
              n188 = call <vilib>:"Check if File or Folder Exists.vi"("path"=w245) -> ("file or folder exists?"=w247:bool, "dup path"=w246:path)  [unwired: 8 in, 1 out]
              n189 = case shown="False" w247 {
                tunnel: w246 -> [w281 w282]
                tunnel: [w280 w282] -> w244
                frame False {
                  n190 = Create Folder(path (use dialog)=w281) -> (created path=w280:path)  [unwired: 2 in, 2 out]
                }
                frame True {
                }
              }
              n191 = Number To Decimal String(number=w260) -> (decimal integer string=w255:string)  [unwired: 1 in]
              n192 = Select(t=w256, s=w258, f=w255) -> (s? t:f=w254:string)
              n193 = Number To Decimal String(number=w259) -> (decimal integer string=w251:string)  [unwired: 1 in]
              n194 = Select(t=w252, s=w261, f=w251) -> (s? t:f=w250:string)
              n195 = call "Build Text2"("T"=w227, "Index"=w265, "Length"=w254, "Width"=w250) -> ("Result"=w249:string)  [unwired: 10 in, 1 out]
              n196 = Build Path(base path=w244, name or relative path=w249) -> (appended path=w262:path)
              n197 = call <vilib>:"Check if File or Folder Exists.vi"("path"=w262) -> ("file or folder exists?"=w264:bool, "dup path"=w263:path)  [unwired: 8 in, 1 out]
              n198 = case shown="True" w264 {
                tunnel: w263 -> [w283 w285]
                tunnel: [w283 w284] -> w228
                frame False {
                }
                frame True {
                  n199 = while {
                    tunnel: w285 -> [w287]
                    tunnel: [w286] -> w284
                    i -> [w289]
                    stop <- w290 stop-if-true
                    n200 = Path To String(path=w287) -> (string=w296:string)
                    n201 = Increment(x=w289) -> (x+1=w288:i32)
                    n202 = Number To Decimal String(number=w288) -> (decimal integer string=w294:string)  [unwired: 1 in]
                    n203 = Concatenate Strings(w296, "_", w294) -> (w293:string)
                    n204 = String To Path(string=w293) -> (path=w292:path)
                    n205 = call <vilib>:"Check if File or Folder Exists.vi"("path"=w292) -> ("file or folder exists?"=w291:bool, "dup path"=w286:path)  [unwired: 8 in, 1 out]
                    n206 = Not(x=w291) -> (.not. x?=w290:bool)
                  }
                }
              }
              n207 = call "transport char run_subvi_2013_04_12_JWa.vi"("VISA session"=w233, "Var1 sweep settings"=w275, "Var2 step settings"=w272, "integration time"=w235, "Path"=w228, "Sample Properties:"=w268) -> ("Graph Cluster"=w226:T21, "error?"=w271:errorcluster)  [unwired: 7 in, 1 out]
              n208 = local write "error out"(w271) -> ()
              n209 = Unbundle By Name(w226) -> ("Transport"=w223:cluster{dbl[], dbl[]}[], "Gate Current"=w222:cluster{dbl[], dbl[]}[])
              n210 = local write "TSP Path"(w228) -> ()
              n211 = Bundle By Name(cluster=w225, "Transport"=w223, "TSP Gate Current"=w222) -> (w224:T4)
              n212 = local write "Graph Cluster"(w224) -> ()
            }
          }
        }
        frame #6 {
          n213 = local write "Status Indicator"(FALSE) -> ()
          n214 = property on="Status Indicator" class="Bool (strict)"("BoolText.Text"="Ready") -> ()  [unwired: 2 in, 2 out]
        }
        frame #7 {
          n215 = disable-structure shown="Disabled" {
            disable-tunnel: w300 -> [w302 _]
            disable-tunnel: w299 -> [w301 _]
            frame Disabled {
              n216 = node-c288(100) -> (w307:T9)  [unwired: 3 in]
              n217 = timed-loop {
                timing: w307 -> [_]
                timing-out: [_] -> w306
                tunnel: w302 -> [w318]
                tunnel: w301 -> [w317]
                tunnel: ["Stop \nCountdown"] -> _
                i -> [w323]
                stop <- w313 stop-if-true
                n218 = node-c288() -> ()  [unwired: 1 in, 1 out]
                n219 = local read "TRF Cluster"() -> (w312:T7)
                n220 = Unbundle By Name(w312) -> ("Loop Wait"=w310:dbl)
                n221 = Multiply(x=0.1, y=w323) -> (x*y=w321:dbl)
                n222 = Equal?(x=w317, y=w318) -> (x = y?=w319:bool)
                n223 = Select(t=0, s=w319, f=w310) -> (s? t:f=w315:dbl)
                n224 = Subtract(x=w315, y=w321) -> (x-y=w309:dbl)
                n225 = Less Or Equal To 0?(x=w309) -> (x <= 0?=w314:bool)
                n226 = Or(x=w314, y="Stop \nCountdown") -> (x .or. y?=w313:bool)
                n227 = Bundle("Loop Wait"=w310, w309) -> (w311:cluster{"Loop Wait":dbl, dbl})  [unwired: 1 in]
                n228 = property on="Status Indicator" class="Bool (strict)"("BoolText.Text"="Waiting...") -> ()  [unwired: 2 in, 2 out]
                n229 = local write "Wait Cluster"(w311) -> ()
                n230 = node-c288() -> ()  [unwired: 1 in, 1 out]
              }
              n231 = node-c288(w306) -> (w303:errorcluster)
              n232 = property on="Status Indicator" class="Bool (strict)"(error in=w303, "BoolText.Text"="Ready") -> ()  [unwired: 1 in, 2 out]
            }
            frame Enabled {
            }
          }
        }
      }
      n233 = local write "VISA resource name out"(w9) -> ()
    }
  }
